vi "Step specific.vi"(10 "Step cluster":T2, 11 "Task condition":string) -> ()   [LabVIEW 2014]
doc: "This VI includes the step name and condition specific code. If a new project is created, this is the main VI to modify."
uses:
  Control/Step name enum.ctl
  <vilib>/Automated Test Systems Ltd/General Tools/Que lib/Write.vi
  <vilib>/Automated Test Systems Ltd/General Tools/Que lib/Que lib.lvlib
panel:
  out "error out":errorcluster
  in  "error in":errorcluster
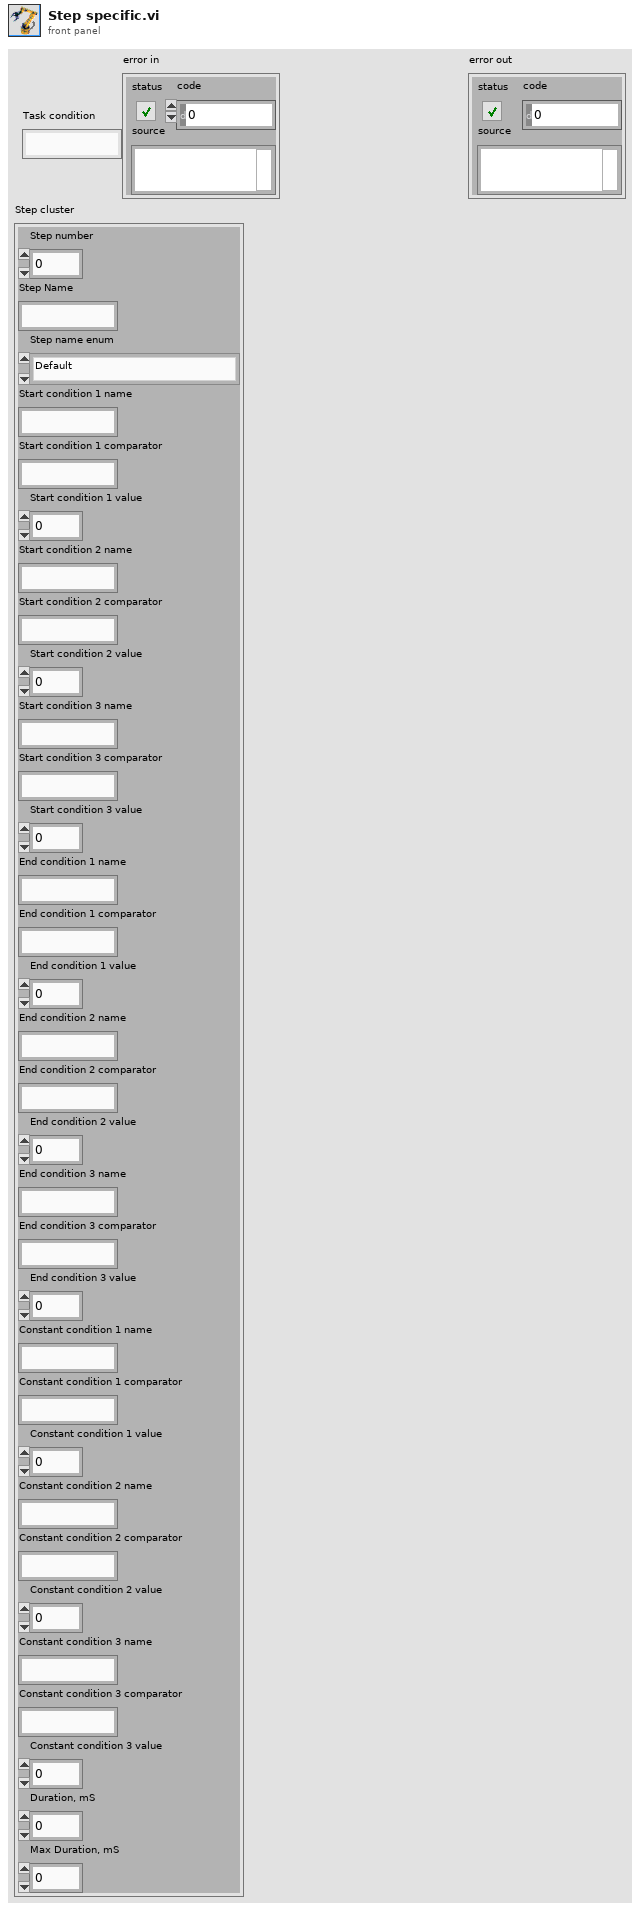
[diagram p1: front panel]
types:
  T1 = typedef "Step name enum.ctl" = enum16{"Default", "Idle", "Init Ard", "Init SM", "Init NI", "Run", "Close"}
  T2 = cluster{"Step number":i32, "Step Name":string, "Step name enum":T1, "Start condition 1 name":string, "Start condition 1 comparator":string, "Start condition 1 value":dbl, "Start condition 2 name":string, "Start condition 2 comparator":string, "Start condition 2 value":dbl, "Start condition 3 name":string, "Start condition 3 comparator":string, "Start condition 3 value":dbl, "End condition 1 name":string, "End condition 1 comparator":string, "End condition 1 value":dbl, "End condition 2 name":string, "End condition 2 comparator":string, "End condition 2 value":dbl, "End condition 3 name":string, "End condition 3 comparator":string, "End condition 3 value":dbl, "Constant condition 1 name":string, "Constant condition 1 comparator":string, "Constant condition 1 value":dbl, "Constant condition 2 name":string, "Constant condition 2 comparator":string, "Constant condition 2 value":dbl, "Constant condition 3 name":string, "Constant condition 3 comparator":string, "Constant condition 3 value":dbl, "Duration, mS":dbl, "Max Duration, mS":dbl}
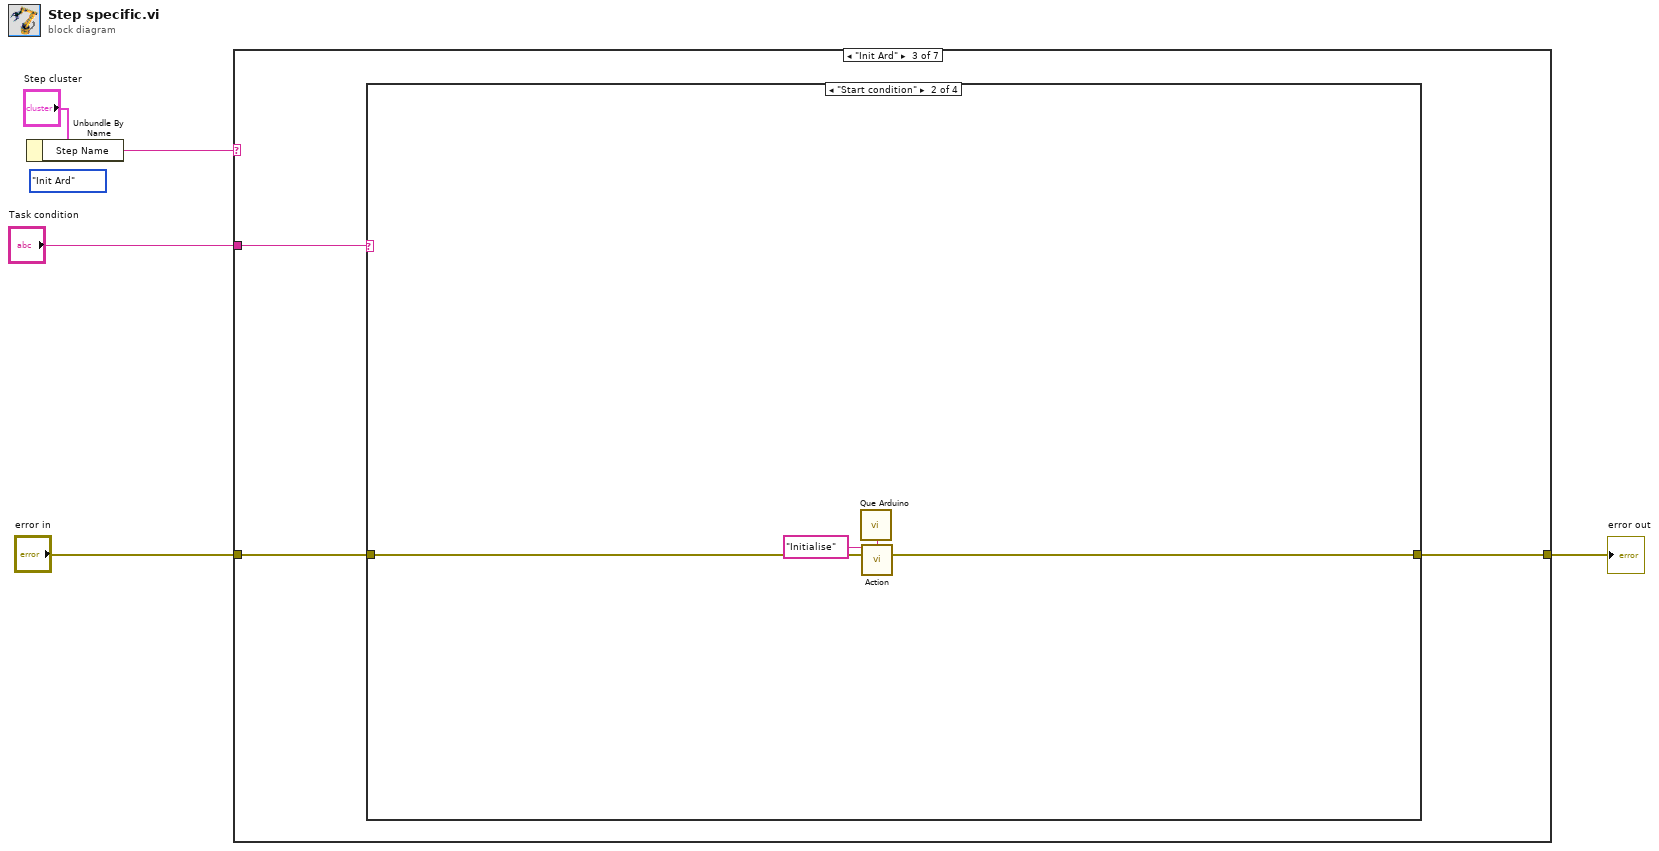
[diagram p0: block diagram]
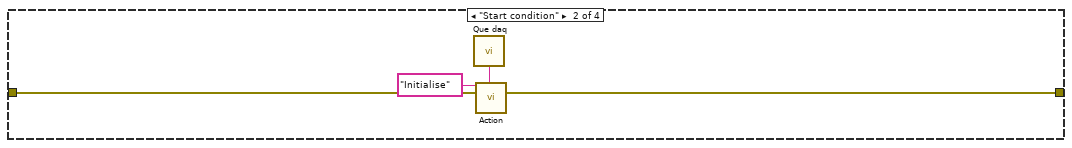
[diagram p12: hidden frame]
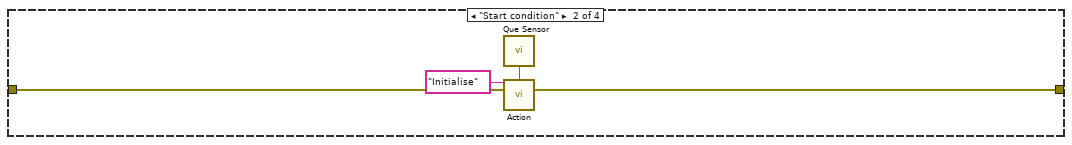
[diagram p16: hidden frame]
diagram:
  (unwired) Step_name_enum."Init Ard" ("Step name enum")
  n1 = Unbundle By Name("Step cluster") -> ("Step Name"=w3:string)
  n2 = case shown="\"Init Ard\"" w3 {
    tunnel: "Task condition" -> [_ w9 w16 w26 w36 w46 w53]
    tunnel: "error in" -> [w6 w7 w15 w25 w35 w45 w51]
    tunnel: [w6 w8 w14 w24 w34 w44 w52] -> w1
    frame "Default", Default {
    }
    frame "Idle" {
      n3 = case shown="\"1\", Default" w9 {
        tunnel: [w10 w11 w12 w13] -> w8
        tunnel: w7 -> [w10 w11 w12 w13]
        frame "1", Default {
        }
        frame "Start" {
        }
        frame "Constant" {
        }
        frame "End" {
        }
      }
    }
    frame "Init Ard" {
      n4 = case shown="\"Start condition\"" w16 {
        tunnel: w15 -> [w17 w20 w22 w23]
        tunnel: [w17 w18 w22 w23] -> w14
        frame "1", Default {
        }
        frame "Start condition" {
          n5 = call <vilib>:"Que Arduino.vi"() -> ("Que name"=w21:string)  [unwired: 15 in]
          n6 = call-poly <vilib>:"Action.vi"("Message"="Initialise", "Que name"=w21, "error in"=w20) -> ("error out"=w18:errorcluster)  [unwired: 12 in]
        }
        frame "Constant condition" {
        }
        frame "End condition" {
        }
      }
    }
    frame "Init NI" {
      n7 = case shown="\"End condition\"" w26 {
        tunnel: w25 -> [w27 w30 w32 w33]
        tunnel: [w27 w28 w32 w33] -> w24
        frame "1", Default {
        }
        frame "Start condition" {
          n8 = call <vilib>:"Que daq.vi"() -> ("Que name"=w29:string)  [unwired: 15 in]
          n9 = call-poly <vilib>:"Action.vi"("Message"="Initialise", "Que name"=w29, "error in"=w30) -> ("error out"=w28:errorcluster)  [unwired: 12 in]
        }
        frame "Constant condition" {
        }
        frame "End condition" {
        }
      }
    }
    frame "Init SM" {
      n10 = case shown="\"End condition\"" w36 {
        tunnel: w35 -> [w37 w40 w42 w43]
        tunnel: [w37 w38 w42 w43] -> w34
        frame "1", Default {
        }
        frame "Start condition" {
          n11 = call <vilib>:"Que Sensor.vi"() -> ("Que name"=w39:string)  [unwired: 15 in]
          n12 = call-poly <vilib>:"Action.vi"("Message"="Initialise", "Que name"=w39, "error in"=w40) -> ("error out"=w38:errorcluster)  [unwired: 12 in]
        }
        frame "Constant condition" {
        }
        frame "End condition" {
        }
      }
    }
    frame "Run" {
      n13 = case shown="\"End condition\"" w46 {
        tunnel: w45 -> [w47 w48 w49 w50]
        tunnel: [w47 w48 w49 w50] -> w44
        frame "1", Default {
        }
        frame "Start condition" {
        }
        frame "Constant condition" {
        }
        frame "End condition" {
        }
      }
    }
    frame "Close" {
      n14 = case shown="\"End condition\"" w53 {
        tunnel: [w54 w55 w56 w57] -> w52
        tunnel: w51 -> [w54 w55 w56 w57]
        frame "1", Default {
        }
        frame "Start condition" {
        }
        frame "Constant condition" {
        }
        frame "End condition" {
        }
      }
    }
  }
  "error out" <- w1
